vi "creat array of dispaly Image.vi"(8 "error in (no error)":errorcluster, 9 "Numeric":u32, 10 "Value":enum16{"1X1", "2X2"}(ring), 11 "CCD monitor in":refnum<class "CCD monitor.lvclass">) -> (0 "error out":errorcluster, 2 "Array":T1[](array[typedef]), 3 "CCD monitor out":refnum<class "CCD monitor.lvclass">)   [LabVIEW 2016, in "Hardware.lvlib" / "CCD monitor.lvlib" / "CCD monitor.lvclass"]
uses:
  <userlib>/Common Components/Hardware/Abstract System/Monitor/CCD monitor.lvclass
  <vilib>/vision/Image Controls.llb/IMAQ Image.ctl
  <userlib>/Common Components/Hardware/CCD/CCD/CCD.lvclass/CCD.ctl
  <userlib>/Common Components/Hardware/Abstract System/Monitor/CCD monitor.lvclass/CCD monitor.ctl
  <userlib>/Common Components/Hardware/CCD/CCD/Read New Image.vi
  <userlib>/Common Components/Hardware/CCD/CCD/CCD.lvclass
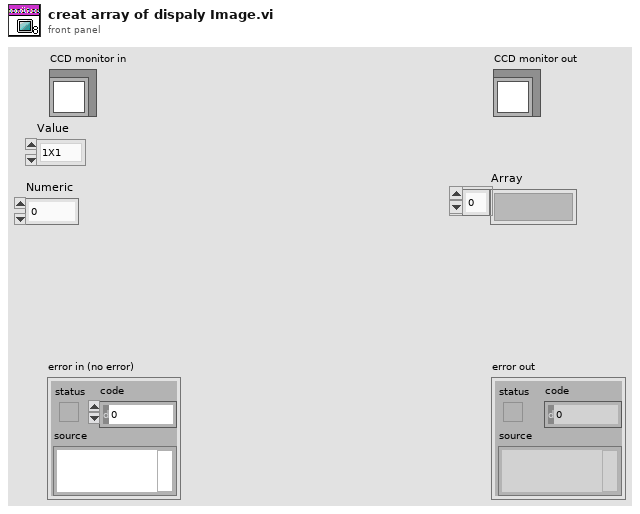
[diagram p1: front panel]
types:
  T1 = typedef "IMAQ Image.ctl" = refnum<image>
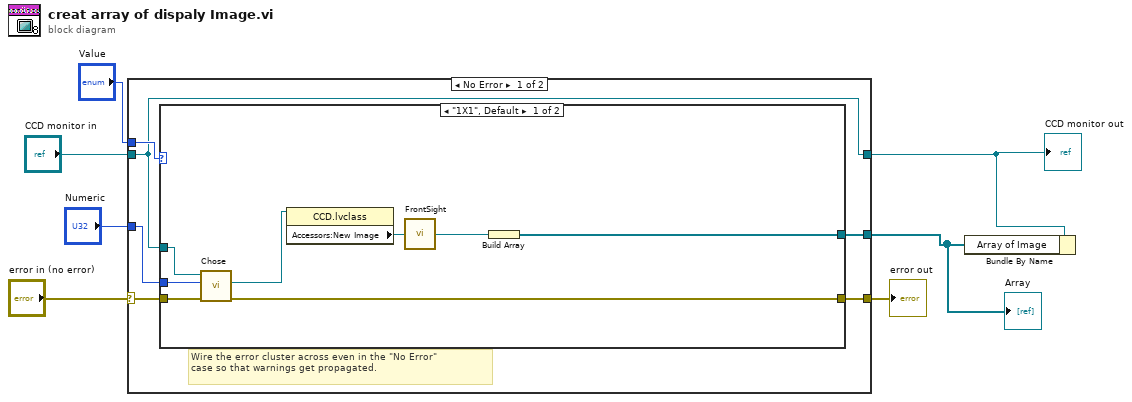
[diagram p0: block diagram]
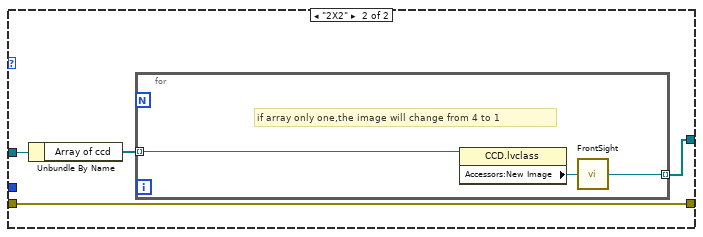
[diagram p2: hidden frame]
diagram:
  n1 = case shown="No Error" "error in (no error)" {
    selector: "error in (no error)" -> [w10 w30]
    tunnel: [w8 w30] -> w6
    tunnel: [w12 w29] -> w2
    tunnel: "CCD monitor in" -> [w12 w29]
    tunnel: "Value" -> [w13 _]
    tunnel: "Numeric" -> [w11 _]
    tunnel: [w9 _] -> w1
    frame No Error {
      # "Wire the error cluster across even in the \"No Error\"\ncase so that warnings get propagated."
      n2 = case shown="\"1X1\", Default" w13 {
        tunnel: w12 -> [w21 w24]
        tunnel: w11 -> [w20 _]
        tunnel: w10 -> [w19 w22]
        tunnel: [w15 w25] -> w9
        tunnel: [w14 w22] -> w8
        frame "1X1", Default {
          n3 = call <userlib>:"Chose.vi"("error in (no error)"=w19, "Numeric"=w20, "CCD monitor in"=w21) -> ("error out"=w14:errorcluster, "element"=w18:refnum<class "CCD.lvclass">)  [unwired: 6 in, 1 out]
          n4 = property class="CCD.lvclass"(reference=w18) -> ("Accessors:New Image"=w17:T1)  [unwired: 1 in, 2 out]
          n5 = call <userlib>:"FrontSight.vi"("IMAQImage"=w17) -> ("Image Out"=w16:T1)
          n6 = Build Array(w16) -> (w15:T1[])
        }
        frame "2X2" {
          n7 = Unbundle By Name(w24) -> ("Array of ccd"=w23:refnum<class "CCD.lvclass">[])
          n8 = for {
            tunnel: [w27] -> w25 mode=indexing
            tunnel: w23 -> [w26] mode=indexing
            # "if array only one,the image will change from 4 to 1"
            n9 = property class="CCD.lvclass"(reference=w26) -> ("Accessors:New Image"=w28:T1)  [unwired: 1 in, 2 out]
            n10 = call <userlib>:"FrontSight.vi"("IMAQImage"=w28) -> ("Image Out"=w27:T1)
          }
        }
      }
    }
    frame Error {
    }
  }
  "error out" <- w6
  "CCD monitor out" <- w2
  "Array" <- w1
  n11 = Bundle By Name(cluster=w2, "Array of Image"=w1) -> ()  [unwired: 1 out]
